vi "SwerveHeadingLock.vi"(3 "Driver Rotation Joystick":dbl, 6 "PID Tuning Parameters":T2={"Kp"=0.0, "Ki"=0.0, "Kd"=0.0, "N-Diff"=10, "N-Int"=10, "Int Error Window"=30.0, "Max Ouput"=1.0, "Min Output"=-1.0} {"Int Error Window" min=0.0; "N-Int" min=2; "N-Diff" min=2; "Kd" min=0.0; "Ki" min=0.0; "Kp" min=0.0}, 8 "Deceleration Hysteresis (ms)":u32, 10 "Heading Lock Strafe Deadband (ft/s)":dbl, 12 "External Disables":bool) -> (14 "Controller Summary":T1(graph), 17 "Joystick Rotation":dbl, 19 "Heading Lock":bool)   [LabVIEW 2019]
uses:
  sensors.vi
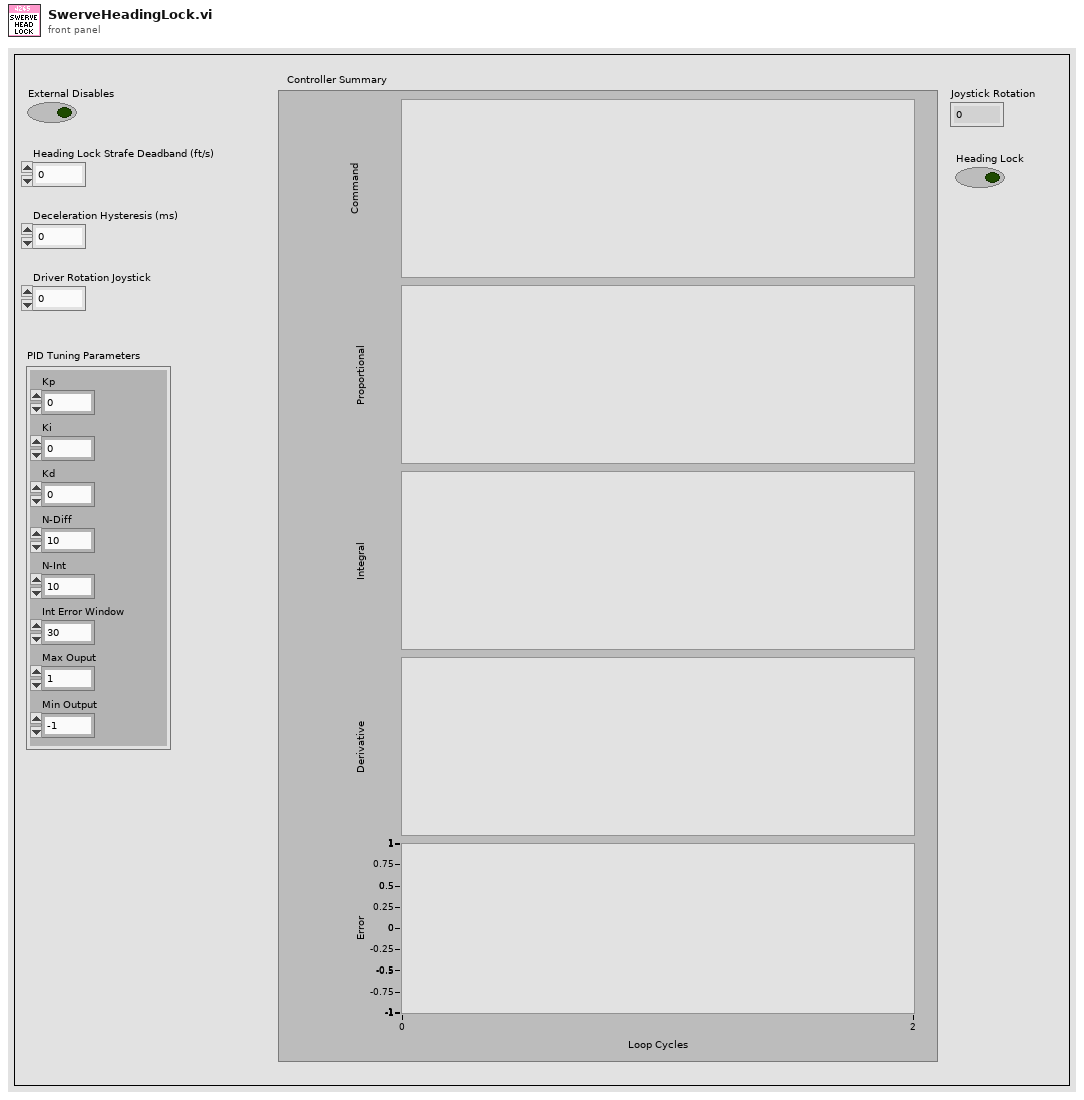
[diagram p1: front panel]
types:
  T1 = cluster{"Command":dbl, "Proportional":dbl, "Integral":dbl, "Derivative":dbl, "Goal":dbl}
  T2 = cluster{"Kp":dbl, "Ki":dbl, "Kd":dbl, "N-Diff":i32, "N-Int":i32, "Int Error Window":dbl, "Max Ouput":dbl, "Min Output":dbl}
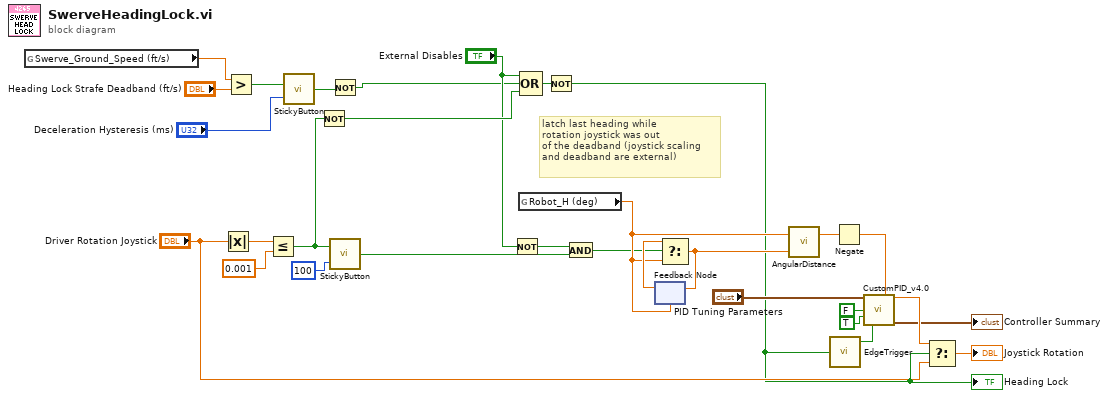
[diagram p0: block diagram]
diagram:
  # "latch last heading while\nrotation joystick was out \nof the deadband (joystick scaling \nand deadband are external)"
  n1 = global read "sensors.vi" "Swerve_Ground_Speed (ft/s)"() -> (w9:dbl)
  n2 = Absolute Value(x="Driver Rotation Joystick") -> (abs(x)=w24:dbl)
  n3 = Greater?(x=w9, y="Heading Lock Strafe Deadband (ft/s)") -> (0:w4:bool)
  n4 = Less Or Equal?(x=w24, y=0.001) -> (x <= y?=w14:bool)
  n5 = call "StickyButton.vi"("Time threshold (ms)"="Deceleration Hysteresis (ms)", "Button Input"=w4) -> ("Sticky Button"=w3:bool)
  n6 = Not(x=w14) -> (.not. x?=w13:bool)
  n7 = Not(x=w3) -> (.not. x?=w2:bool)
  n8 = call "StickyButton.vi"("Time threshold (ms)"=u32 100 ("y"), "Button Input"=w14) -> ("Sticky Button"=w8:bool)
  n9 = Not(x="External Disables") -> (.not. x?=w6:bool)
  n10 = global read "sensors.vi" "Robot_H (deg)"() -> (w15:dbl)
  n11 = Compound Arithmetic op=OR("External Disables", w2, w13) -> (w12:bool)
  n12 = Not(x=w12) -> (.not. x?=w11:bool)
  "Heading Lock" <- w11
  n13 = And(x=w6, y=w8) -> (x .and. y?=w5:bool)
  n14 = feedback #1(w15) -> (w16:dbl)
  n15 = Select(t=w16, s=w5, f=w15) -> (s? t:f=w25:dbl)
  n16 = feedback-in #1(w25) -> ()
  n17 = call "AngularDistance.vi"("Goal Angle (deg) [0,360]"=w25, "Current Angle (deg) [-Inf,+Inf]"=w15) -> ("Signed Angular Distance (deg) [-180,+180]"=w23:dbl)  [unwired: 1 out]
  n18 = call "EdgeTrigger.vi"("Input Signal"=w11) -> ("Rising Edge Trigger"=w28:bool)  [unwired: 2 out]
  n19 = Negate(x=w23) -> (-x=w26:dbl)
  n20 = call "CustomPID_v4.0.vi"("PID Tuning Parameters"="PID Tuning Parameters", "Custom Error Calculation"=w26, "Reset on Goal Change ?"=FALSE, "Use Custom Error Calculation ?"=TRUE, "Reinit"=w28) -> ("Command"=w22:dbl, "Controller Summary"=→"Controller Summary":T1)  [unwired: 7 in, 2 out]
  n21 = Select(t=w22, s=w11, f="Driver Rotation Joystick") -> (s? t:f=→"Joystick Rotation":dbl)
